vi "addDataU8.vi"(8 "error in (no error)":errorcluster, 10 "Data":u8, 11 "DynamicFrameBuilder in":refnum<class "DynamicFrameBuilder.lvclass">) -> (0 "error out":errorcluster, 3 "DynamicFrameBuilder out":refnum<class "DynamicFrameBuilder.lvclass">)   [LabVIEW 2016, in "RTModbus.lvlib" / "DynamicFrameBuilder.lvclass"]
uses:
  DynamicFrameBuilder.lvclass
  DynamicFrameBuilder.lvclass/DynamicFrameBuilder.ctl
  Common_RT_Utilities/U8ArrayBuilderAutoIndexing/U8ArrayBuilderAutoIndexing.lvclass
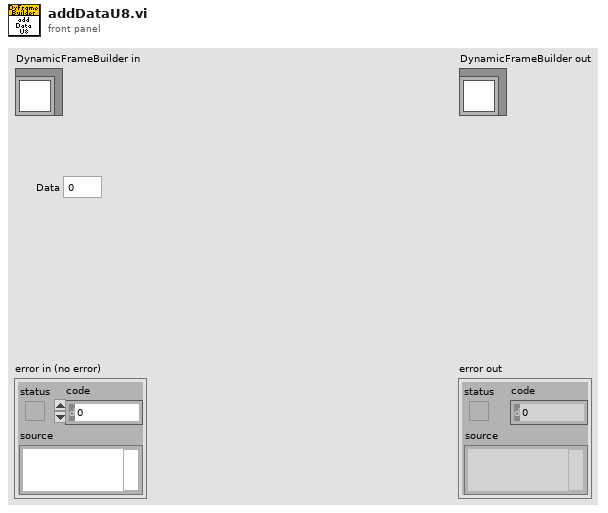
[diagram p1: front panel]
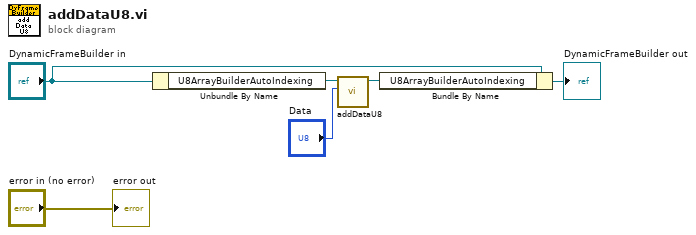
[diagram p0: block diagram]
diagram:
  n1 = Unbundle By Name("DynamicFrameBuilder in") -> ("U8ArrayBuilderAutoIndexing"=w3:refnum<class "U8ArrayBuilderAutoIndexing.lvclass">)
  n2 = call "addDataU8.vi"("Data"="Data", "U8ArrayBuilderAutoIndexing in"=w3) -> ("U8ArrayBuilderAutoIndexing out"=w1:refnum<class "U8ArrayBuilderAutoIndexing.lvclass">)  [unwired: 8 in, 1 out]
  n3 = Bundle By Name(cluster="DynamicFrameBuilder in", "U8ArrayBuilderAutoIndexing"=w1) -> (→"DynamicFrameBuilder out":refnum<class "DynamicFrameBuilder.lvclass">)
  "error out" <- "error in (no error)"
